vi "Get Proj Item Ref from Lib Name.vi"(0 "ProjectItem in":refnum<vi>, 5 "LIbrary Name":string, 11 "error in (no error)":errorcluster) -> (4 "ProjectItem out":refnum<vi>, 6 "Found":bool, 15 "error out":errorcluster)   [LabVIEW 2019, in "MVA Message Mapper.lvlib"]
uses:
  <vilib>/gpm_packages/@cs/Bus-message-mapper/Source/MVA Message Mapper.lvlib
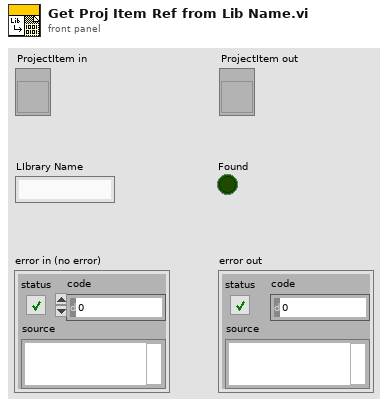
[diagram p1: front panel]
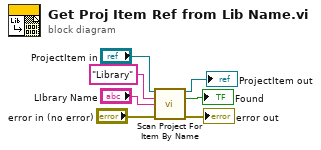
[diagram p0: block diagram]
diagram:
  n1 = call <vilib>:"Scan Project For Item By Name.vi"("ProjectItem in"="ProjectItem in", "Type"="Library", "Item Name"="LIbrary Name", "error in (no error)"="error in (no error)") -> ("ProjectItem out"=→"ProjectItem out":refnum<vi>, "Found"=→"Found":bool, "error out"=→"error out":errorcluster)  [unwired: 9 in]
